vi "Pocess rprfrq.vi"(8 "error in (no error)":errorcluster, 9 "Plot in":cluster{dbl[], dbl[]}[](array[cluster]), 10 "Result in":refnum<class "Acquired Result.lvclass">, 11 "Elastic Moduli in":refnum<class "Elastic Moduli.lvclass">) -> (0 "error out":errorcluster, 1 "Plot out":cluster{dbl[], dbl[]}[](array[cluster]), 2 "Result out":refnum<class "Acquired Result.lvclass">, 3 "Elastic Moduli out":refnum<class "Elastic Moduli.lvclass">)   [LabVIEW 2016, in "Elastic Moduli.lvclass"]
uses:
  Elastic Moduli.lvclass
  NHMFL_Core/Libraries/Instruments/Results/Acquired Result/Acquired Result.lvclass
  <vilib>/Utility/file.llb/Read Delimited Spreadsheet (DBL).vi
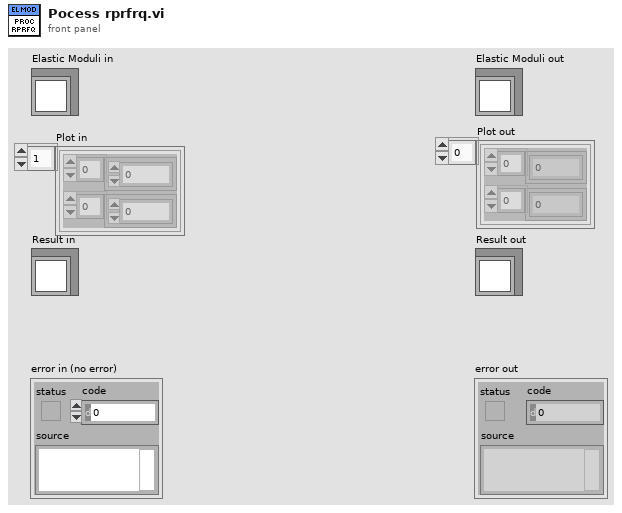
[diagram p1: front panel]
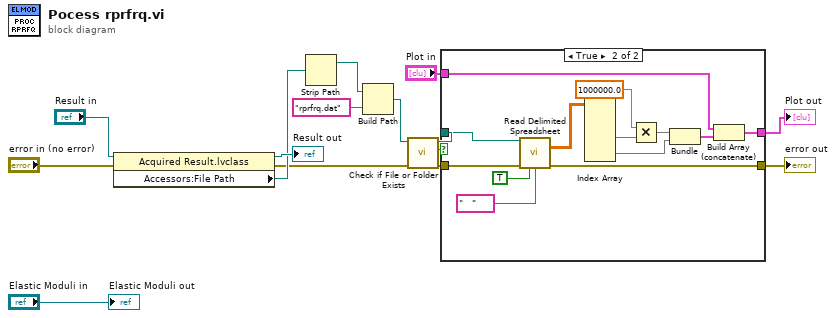
[diagram p0: block diagram]
diagram:
  n1 = property class="Acquired Result.lvclass"(reference="Result in", error in="error in (no error)") -> (reference out=→"Result out":refnum<class "Acquired Result.lvclass">, error out=w7:errorcluster, "Accessors:File Path"=w9:path)
  n2 = Strip Path(path=w9) -> (stripped path=w10:path)  [unwired: 1 out]
  n3 = Build Path(base path=w10, name or relative path="rprfrq.dat") -> (appended path=w8:path)
  n4 = call <vilib>:"Check if File or Folder Exists.vi"("error in (no error)"=w7, "path"=w8) -> ("error out"=w4:errorcluster, "file or folder exists?"=w6:bool, "dup path"=w5:path)  [unwired: 7 in]
  n5 = case shown="True" w6 {
    tunnel: w5 -> [_ w30]
    tunnel: w4 -> [w16 w29]
    tunnel: "Plot in" -> [w17 w25]
    tunnel: [w17 w24] -> w2
    tunnel: [w16 w23] -> w1
    frame False {
    }
    frame True {
      n6 = call-poly <vilib>:"Read Delimited Spreadsheet.vi"("file path (dialog if empty)"=w30, "error in (no error)"=w29, "transpose? (F)"=TRUE, "delimiter (\\t)"="   " ("delimiter (\\t)")) -> ("all rows"=w28:dbl[][], "error out"=w23:errorcluster)  [unwired: 6 in, 4 out]
      n7 = Index Array(array=w28) -> (element #2=w20:dbl[], element #3=w26:dbl[])  [unwired: 6 in, 1 out]
      n8 = Multiply(x=1000000.0, y=w20) -> (x*y=w21:dbl[])
      n9 = Bundle(w21, "all rows"=w26) -> (w27:cluster{dbl[], "all rows":dbl[]})  [unwired: 1 in]
      n10 = Build Array (concatenate)(w25, w27) -> (w24:cluster{dbl[], "all rows":dbl[]}[])
    }
  }
  "error out" <- w1
  "Plot out" <- w2
  "Elastic Moduli out" <- "Elastic Moduli in"
